vi "2D Polynomial Evaluation (CDB).vi"(2 "P(x)":cdb[](array[numeric]), 3 "A":cdb[][](array[numeric])) -> (0 "error":i32, 1 "P(A)":cdb[][](array[numeric]))   [LabVIEW 2020, in "NI_AALPro.lvlib"]
doc: "Evaluates the polynomial <B>P(x)</B> with a single value or multiple values. The data types you wire to the <B>a</B> and <B>P(x)</B> inputs determine the polymorphic instance to use."
uses:
  <vilib>/Analysis/NI_AALPro.lvlib
  <vilib>/Analysis/polynomials.llb/Remove Zero Coefficients (CDB).vi
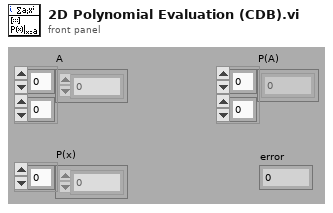
[diagram p1: front panel]
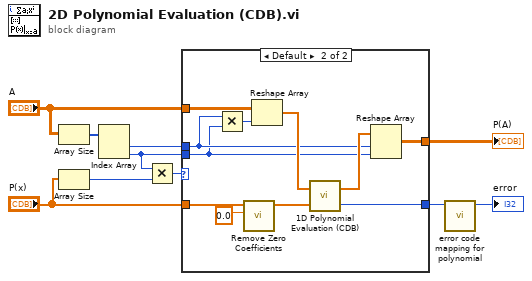
[diagram p0: block diagram]
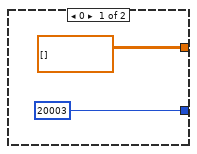
[diagram p2: hidden frame]
diagram:
  n1 = Array Size(array="A") -> (size(s)=w8:i32[])
  n2 = Array Size(array="P(x)") -> (size(s)=w6:i32)
  n3 = Index Array(array=w8) -> (element #1=w3:i32, element #2=w4:i32)  [unwired: 2 in]
  n4 = Multiply(x=w4, y=w6) -> (x*y=w7:i32)
  n5 = case shown="Default" w7 {
    tunnel: "P(x)" -> [_ w22]
    tunnel: [cdb[][] [] w13] -> w10
    tunnel: [20003 ("empty array") w17] -> w2
    tunnel: "A" -> [_ w19]
    tunnel: w4 -> [_ w14]
    tunnel: w3 -> [_ w15]
    frame 0 {
    }
    frame Default {
      n6 = Multiply(x=w15, y=w14) -> (x*y=w20:i32)
      n7 = call-poly <vilib>:"Remove Zero Coefficients.vi"("threshold"=0.0, "P(x) In"=w22) -> ("P(x) Out"=w21:cdb[])  [unwired: 7 in, 2 out]
      n8 = Reshape Array(w19, w20) -> (w18:cdb[])
      n9 = call <vilib>:"1D Polynomial Evaluation (CDB).vi"("P(x)"=w21, "A"=w18) -> ("error"=w17:i32, "P(A)"=w16:cdb[])
      n10 = Reshape Array(w16, w15, w14) -> (w13:cdb[][])
    }
  }
  "P(A)" <- w10
  n11 = call <vilib>:"error code mapping for polynomial.vi"("error in"=w2) -> ("error out"=→"error":i32)  [unwired: 10 in]
